vi "Read PID gains.vi"(8 "error in (no error)":errorcluster, 11 "PID Loop in":refnum<class "PID Loop.lvclass">) -> (0 "error out":errorcluster, 2 "PID gains":T1={"proportional gain (Kc)"=1.0, "integral time (Ti, min)"=0.01, "derivative time (Td, min)"=0.0} {"proportional gain (Kc)" format="%.2f"; "integral time (Ti, min)" format="%.2f"}, 3 "PID Loop out":refnum<class "PID Loop.lvclass">)   [LabVIEW 2013, in "PID Loop.lvclass"]
uses:
  PID Loop.lvclass
  PID Gains.ctl
  PID Loop.lvclass/PID Loop.ctl
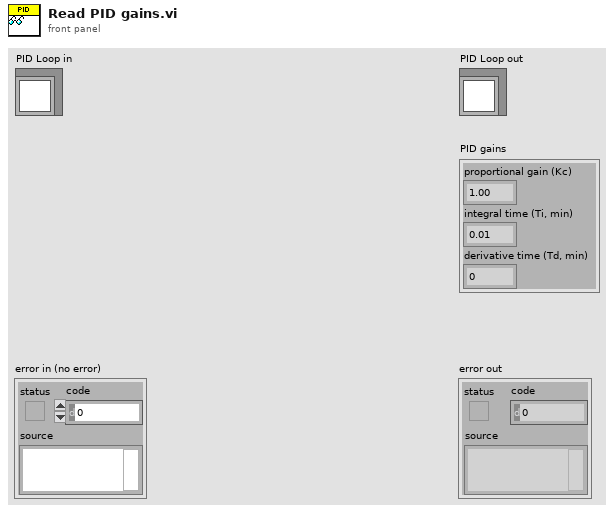
[diagram p1: front panel]
types:
  T1 = typedef "PID Loop.lvclass/PID Gains.ctl" = cluster{"proportional gain (Kc)":dbl, "integral time (Ti, min)":dbl, "derivative time (Td, min)":dbl}
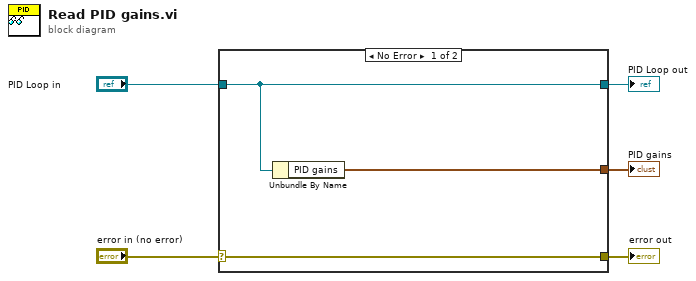
[diagram p0: block diagram]
diagram:
  n1 = case shown="No Error" "error in (no error)" {
    selector: "error in (no error)" -> [w8 w9]
    tunnel: [w8 w9] -> w4
    tunnel: [w7 w10] -> w2
    tunnel: "PID Loop in" -> [w7 w10]
    tunnel: [w6 _] -> w1
    frame No Error {
      n2 = Unbundle By Name(w7) -> ("PID gains"=w6:T1)
    }
    frame Error {
    }
  }
  "error out" <- w4
  "PID Loop out" <- w2
  "PID gains" <- w1
